vi "GetFlags.vi"(8 "error in (no error)":errorcluster, 11 "C37.118FlagImpairPlugin in":refnum<class "C37.118FlagImpairPlugin.lvclass">) -> (0 "error out":errorcluster, 3 "C37.118FlagImpairPlugin out":refnum<class "C37.118FlagImpairPlugin.lvclass">)   [LabVIEW 2017, in "FlagImpairPlugins.lvlib" / "C37.118FlagImpairPlugin.lvclass"]
uses:
  C37.118FlagImpairPlugin.lvclass
  C:/dev/Work/PARTF/Modules/FlagImpairPlugins/FlagImpairPluginBase_class/FlagImpairPluginBase.lvclass
  FlagImpairPluginBase_class/Accessors/Read clFlagImpairConfig.vi
  FlagImpairPluginBase_class/Accessors/Read FlagImpairParams.vi
  FlagImpairPluginBase_class/Accessors/Read TimeArray.vi
  FlagImpairPluginBase_class/Accessors/Set FlagImpairmentArray.vi
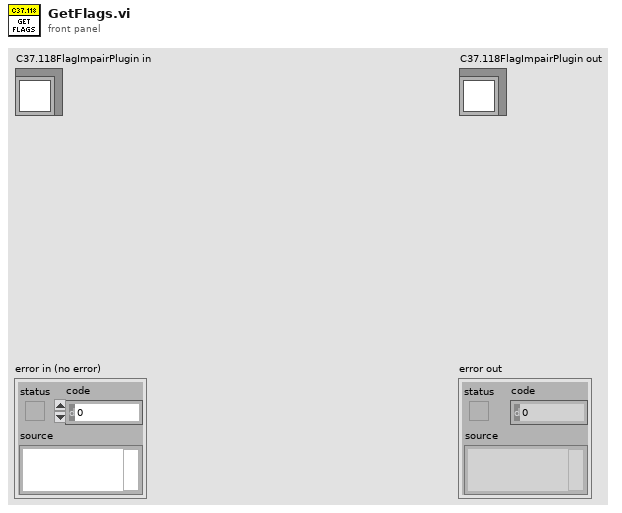
[diagram p1: front panel]
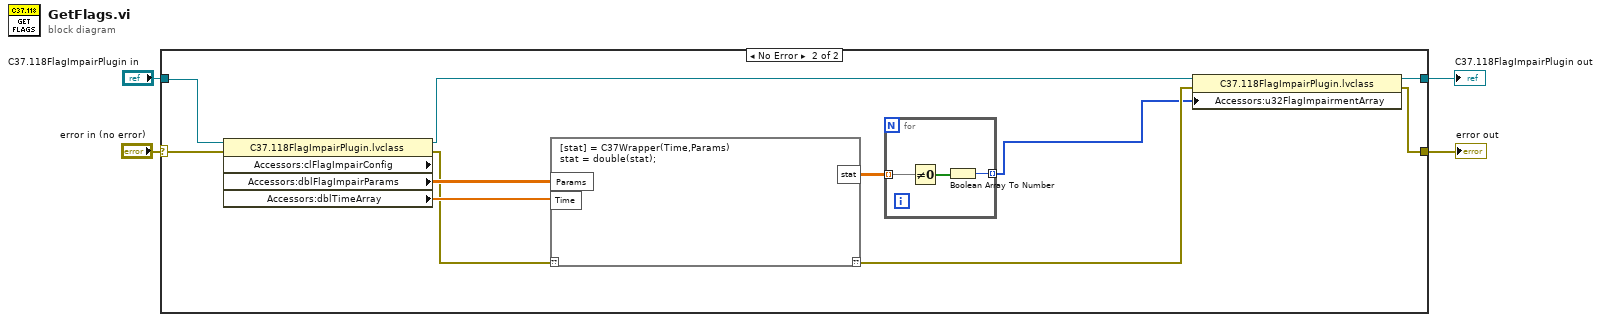
[diagram p0: block diagram]
diagram:
  n1 = case shown="No Error" "error in (no error)" {
    selector: "error in (no error)" -> [w6 w14]
    tunnel: [w5 w17] -> w2
    tunnel: "C37.118FlagImpairPlugin in" -> [w5 w15]
    tunnel: [w6 w16] -> w1
    frame Error {
    }
    frame No Error {
      n2 = property class="C37.118FlagImpairPlugin.lvclass" props=["Accessors:clFlagImpairConfig", "Accessors:dblFlagImpairParams", "Accessors:dblTimeArray"](reference=w15, error in=w14) -> (reference out=w13:refnum<class "C37.118FlagImpairPlugin.lvclass">, error out=w9:errorcluster, "Accessors:dblFlagImpairParams"=w11:dbl[][], "Accessors:dblTimeArray"=w10:dbl[])  [unwired: 1 out]
      n3 = script code="[stat] = C37Wrapper(Time,Params)\nstat = double(stat);"("??"=w9, "Params"=w11, "Time"=w10) -> ("??"=w12:errorcluster, "stat"=w7:dbl[][])
      n4 = for {
        tunnel: w7 -> [w19] mode=indexing
        tunnel: [w20] -> w8 mode=indexing
        n5 = Not Equal To 0?(x=w19) -> (x != 0?=w18:bool[])
        n6 = Boolean Array To Number(Boolean array=w18) -> (number=w20:u32)
      }
      n7 = property class="C37.118FlagImpairPlugin.lvclass"(reference=w13, error in=w12, "Accessors:u32FlagImpairmentArray"=w8) -> (reference out=w17:refnum<class "C37.118FlagImpairPlugin.lvclass">, error out=w16:errorcluster)
    }
  }
  "error out" <- w1
  "C37.118FlagImpairPlugin out" <- w2
